vi "Zero.vi"(8 "error in (no error)":errorcluster, 11 "VISA resource name":refnum<visa-resource-name>) -> (0 "error out":errorcluster, 3 "VISA resource name out":refnum<visa-resource-name>)   [LabVIEW 2015, in "Ohaus AV Series.lvlib"]
doc: "This VI zeroes the balance."
uses:
  Ohaus AV Series.lvlib
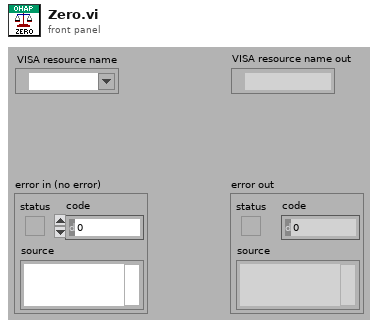
[diagram p1: front panel]
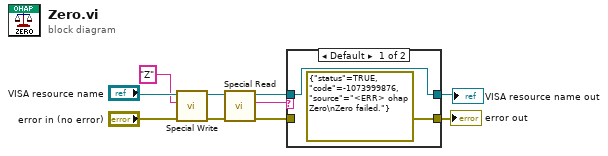
[diagram p0: block diagram]
diagram:
  n1 = call "Special Write.vi"("error in (no error)"="error in (no error)", "Input String"="Z", "VISA resource name"="VISA resource name") -> ("error out"=w8:errorcluster, "VISA resource name out"=w9:refnum<visa-resource-name>)  [unwired: 7 in]
  n2 = call "Special Read.vi"("error in (no error)"=w8, "VISA resource name"=w9) -> ("error out"=w3:errorcluster, "Output String"=w2:string, "VISA resource name out"=w4:refnum<visa-resource-name>)  [unwired: 7 in]
  n3 = case shown="Default" w2 {
    tunnel: [errorcluster {"status"=TRUE, "code"=-1073999876, "source"="<ERR> ohap Zero\nZero failed."} ("error out") w14] -> w10
    tunnel: w4 -> [w11 w13]
    tunnel: w3 -> [_ w14]
    tunnel: [w11 w13] -> w1
    frame Default {
    }
    frame "OK!\r\n" {
    }
  }
  "error out" <- w10
  "VISA resource name out" <- w1
